vi "Load Cell Multiplier.vi"() -> ()   [LabVIEW 2012]
panel:
  in  "Load Cell Multiplier":dbl
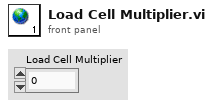
[diagram p1: front panel]
diagram:
